vi "PathPlanner_PathFinder_Heuristic.vi"(9 "sGoalLoc":T1, 11 "sStartLoc":T1) -> (3 "heuristic":dbl)   [LabVIEW 2019]
uses:
  PathPlannerLib24/TypeDef/PathPlannerFinderGridPosition.ctl
  PathPlannerLib24/PathPlanner24.lvlib
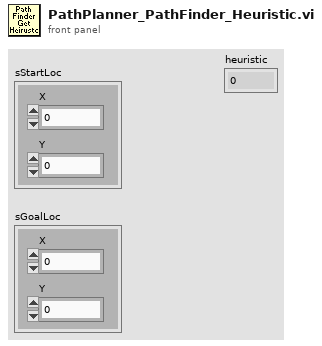
[diagram p1: front panel]
types:
  T1 = typedef "PathPlanner24.lvlib/PathPlannerFinderGridPosition.ctl" = cluster{"X":i32, "Y":i32}
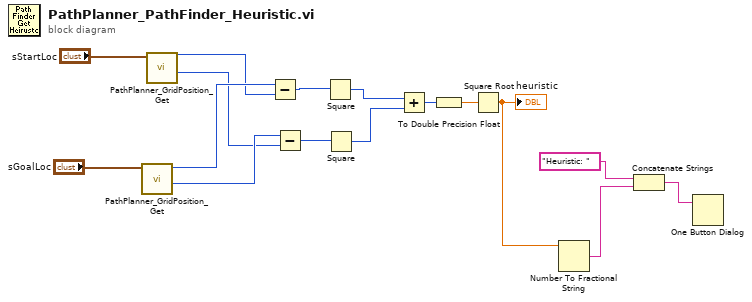
[diagram p0: block diagram]
diagram:
  n1 = call "PathPlanner_GridPosition_Get.vi"("GridPosition"="sGoalLoc") -> ("Int Y"=w12:i32, "Int X"=w14:i32)  [unwired: 9 in]
  n2 = call "PathPlanner_GridPosition_Get.vi"("GridPosition"="sStartLoc") -> ("Int Y"=w11:i32, "Int X"=w13:i32)  [unwired: 9 in]
  n3 = Subtract(x=w14, y=w13) -> (x-y=w7:i32)
  n4 = Subtract(x=w12, y=w11) -> (x-y=w8:i32)
  n5 = Square(x=w7) -> (x^2=w6:i32)
  n6 = Square(x=w8) -> (x^2=w5:i32)
  n7 = Add(x=w6, y=w5) -> (x+y=w10:i32)
  n8 = To Double Precision Float(number=w10) -> (double precision float=w9:dbl)
  n9 = Square Root(x=w9) -> (sqrt(x)=w4:dbl)
  "heuristic" <- w4
  n10 = Number To Fractional String(number=w4) -> (F-format string=w3:string)  [unwired: 3 in]
  n11 = Concatenate Strings("Heuristic: " ("string"), w3) -> (w1:string)
  n12 = One Button Dialog(message=w1) -> ()  [unwired: 1 in, 1 out]
